vi "Check for wavelength or frequency errors.vi"(8 "error in (no error)":errorcluster, 10 "F or lambda in":dbl) -> (0 "error out":errorcluster, 2 "F or lambda out":dbl)   [LabVIEW 2009]
doc: "Takes the result of a 'get' operation on the wavelength meter and checks for errors."
uses:
  <vilib>/Utility/error.llb/DialogType.ctl
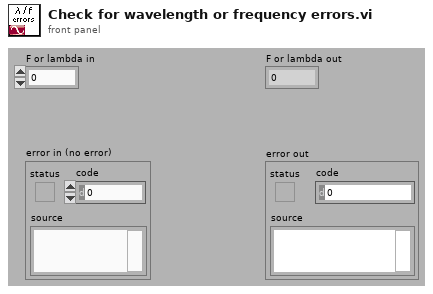
[diagram p1: front panel]
types:
  T1 = typedef "DialogType.ctl" = u16
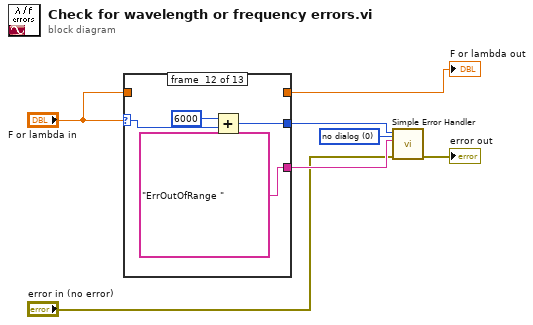
[diagram p0: block diagram]
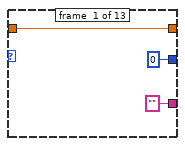
[diagram p2: hidden frame]
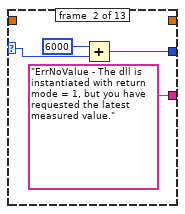
[diagram p3: hidden frame]
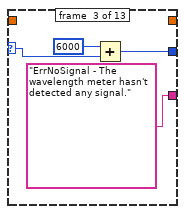
[diagram p4: hidden frame]
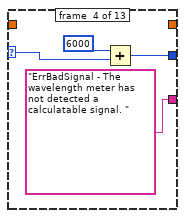
[diagram p5: hidden frame]
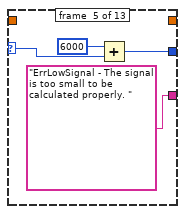
[diagram p6: hidden frame]
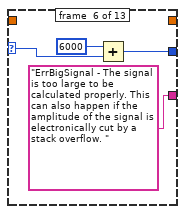
[diagram p7: hidden frame]
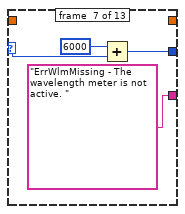
[diagram p8: hidden frame]
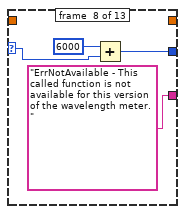
[diagram p9: hidden frame]
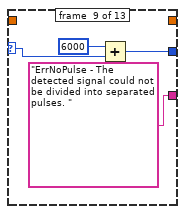
[diagram p10: hidden frame]
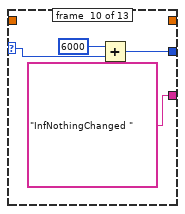
[diagram p11: hidden frame]
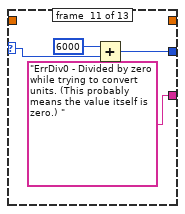
[diagram p12: hidden frame]
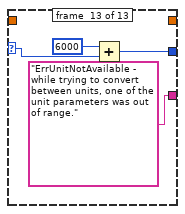
[diagram p13: hidden frame]
diagram:
  w7 = T1 0 items=["no dialog", "OK message", "continue or stop message", "OK message + warnings", "continue/stop + warnings"] ("type of dialog (OK msg:1)")
  n1 = case shown="Default" "F or lambda in" {
    selector: "F or lambda in" -> [_ w13 w16 w20 w24 w28 w32 w35 w40 w43 w47 w51 w56]
    tunnel: ["" ("error source (\" \")") "ErrNoValue - The dll is instantiated with return mode = 1, but you have requested the latest measured value." ("error source (\" \")") "ErrNoSignal - The wavelength meter hasn't detected any signal." ("error source (\" \")") "ErrBadSignal - The wavelength meter has not detected a calculatable signal. " ("error source (\" \")") "ErrLowSignal - The signal is too small to be calculated properly. " ("error source (\" \")") "ErrBigSignal - The signal is too large to be calculated properly. This can also happen if the amplitude of the signal is electronically cut by a stack overflow. " ("error source (\" \")") "ErrWlmMissing - The wavelength meter is not active. " ("error source (\" \")") "ErrNotAvailable - This called function is not available for this version of the wavelength meter. " ("error source (\" \")") "ErrNoPulse - The detected signal could not be divided into separated pulses. " ("error source (\" \")") "InfNothingChanged " ("error source (\" \")") "ErrDiv0 - Divided by zero while trying to convert units. (This probably means the value itself is zero.) " ("error source (\" \")") "ErrOutOfRange " ("error source (\" \")") "ErrUnitNotAvailable - while trying to convert between units, one of the unit parameters was out of range." ("error source (\" \")")] -> w6
    tunnel: [0 w11 w15 w19 w23 w27 w31 w36 w39 w44 w48 w52 w55] -> w3
    tunnel: "F or lambda in" -> [w8 _ _ _ _ _ _ _ _ _ _ _ _]
    tunnel: [w8 _ _ _ _ _ _ _ _ _ _ _ _] -> w1
    frame #0 {
    }
    frame #1 {
      n2 = Add(x=6000, y=w13) -> (x+y=w11:i32)
    }
    frame #2 {
      n3 = Add(x=6000, y=w16) -> (x+y=w15:i32)
    }
    frame #3 {
      n4 = Add(x=6000, y=w20) -> (x+y=w19:i32)
    }
    frame #4 {
      n5 = Add(x=6000, y=w24) -> (x+y=w23:i32)
    }
    frame #5 {
      n6 = Add(x=6000, y=w28) -> (x+y=w27:i32)
    }
    frame #6 {
      n7 = Add(x=6000, y=w32) -> (x+y=w31:i32)
    }
    frame #7 {
      n8 = Add(x=6000, y=w35) -> (x+y=w36:i32)
    }
    frame #8 {
      n9 = Add(x=6000, y=w40) -> (x+y=w39:i32)
    }
    frame #9 {
      n10 = Add(x=6000, y=w43) -> (x+y=w44:i32)
    }
    frame #10 {
      n11 = Add(x=6000, y=w47) -> (x+y=w48:i32)
    }
    frame #11 {
      n12 = Add(x=6000, y=w51) -> (x+y=w52:i32)
    }
    frame #12 {
      n13 = Add(x=6000, y=w56) -> (x+y=w55:i32)
    }
  }
  "F or lambda out" <- w1
  n14 = call <vilib>:"Simple Error Handler.vi"("error code (no error:0)"=w3, "error source (\" \")"=w6, "type of dialog (OK msg:1)"=w7, "error in (no error)"="error in (no error)") -> ("error out"=→"error out":errorcluster)  [unwired: 5 out]
